vi "Execute.vi"(8 "error in":errorcluster, 9 "Consumer Queues in":T1, 10 "DAC Process Command in":refnum<class "Stop DAC.lvclass">, 11 "DAC Process Data in":T2) -> (0 "error out":errorcluster, 1 "Consumer Queues out":T1, 2 "Stop?":bool, 3 "DAC Process Data out":T2)   [LabVIEW 2019, in "DAC Process.lvlib" / "Stop DAC.lvclass"]
uses:
  Stop DAC.lvclass
  DAC Process Data.ctl
  Generic Test Stand/Generic Test Stand.lvclass
  TS Framework/ExeLogging/DAC Logger/DAC Logger.lvclass
  DAC State.ctl
  TS Framework/Consumer Queues.ctl
  UI Process/Generic UI Command/Generic UI Process Command.lvclass
  Generic DAC Command/Generic DAC Process Command.lvclass
  Trig Process/Generic Trig Command/Generic Trig Process Command.lvclass
  UI Process/UI Idle State/UI Idle State.lvclass
  Generic Test Stand/Generic Test Stand.lvclass/Generic Test Stand.ctl
  DAC Process.lvlib
  TS Framework/TS Framework.lvlib
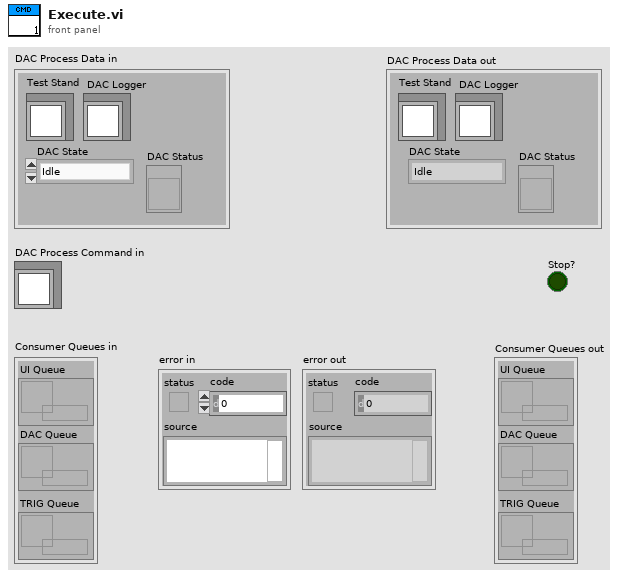
[diagram p1: front panel]
types:
  T1 = typedef "TS Framework.lvlib/Consumer Queues.ctl" = cluster{"UI Queue":refnum<queue>, "DAC Queue":refnum<queue>, "TRIG Queue":refnum<queue>}
  T2 = typedef "DAC Process.lvlib/DAC Process Data.ctl" = cluster{"Test Stand":refnum<class "Generic Test Stand.lvclass">, " DAC Logger":refnum<class "DAC Logger.lvclass">, "DAC State":T3, "DAC Status":refnum<vi>}
  T3 = typedef "DAC Process.lvlib/DAC State.ctl" = enum16{"Idle", "Acquiring"}
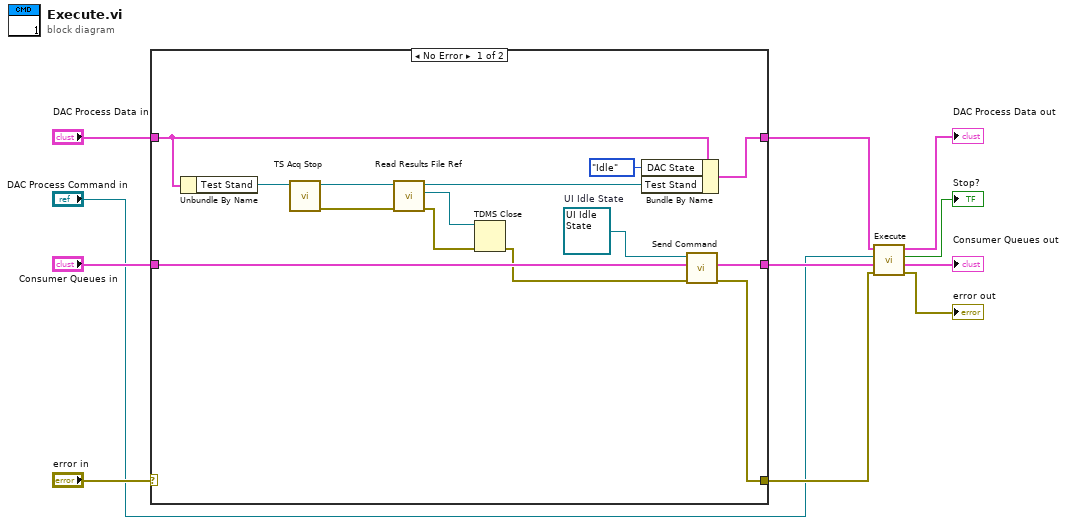
[diagram p0: block diagram]
diagram:
  n1 = case shown="No Error" "error in" {
    selector: "error in" -> [_ w28]
    tunnel: [w20 w28] -> w2
    tunnel: "DAC Process Data in" -> [w17 w27]
    tunnel: [w24 w27] -> w6
    tunnel: "Consumer Queues in" -> [w23 w26]
    tunnel: [w21 w26] -> w3
    frame No Error {
      w22 = refnum<class "UI Idle State.lvclass"> refnum  # UI Idle State
      n2 = Unbundle By Name(w17) -> ("Test Stand"=w15:refnum<class "Generic Test Stand.lvclass">)
      n3 = call-dynamic "TS Acq Stop.vi"("Generic Test Stand in"=w15) -> ("error out"=w13:errorcluster, "Generic Test Stand out"=w14:refnum<class "Generic Test Stand.lvclass">)  [unwired: 9 in]
      n4 = call "Read Results File Ref.vi"("error in (no error)"=w13, "Generic Test Stand in"=w14) -> ("error out"=w18:errorcluster, "Results File Ref"=w19:refnum<k34>, "Generic Test Stand out"=w12:refnum<class "Generic Test Stand.lvclass">)  [unwired: 7 in]
      n5 = TDMS Close(8:w18, 11:w19) -> (0:w16:errorcluster)  [unwired: 1 out]
      n6 = Bundle By Name(cluster=w17, "DAC State"=DAC_State."Idle", "Test Stand"=w12) -> (w24:T2)
      n7 = call-dynamic "Send Command.vi"("error in (no error)"=w16, "Consumer Queues in"=w23, "UI Process Command in"=w22) -> ("error out"=w20:errorcluster, "Consumer Queues out"=w21:T1)  [unwired: 7 in]
    }
    frame Error {
    }
  }
  n8 = call-parent "Execute.vi"("error in"=w2, "Consumer Queues in"=w3, "DAC Process Command in"="DAC Process Command in", "DAC Process Data in"=w6) -> ("error out"=→"error out":errorcluster, "Consumer Queues out"=→"Consumer Queues out":T1, "Stop?"=→"Stop?":bool, "DAC Process Data out"=→"DAC Process Data out":T2)  [unwired: 4 in]
